vi "testevent.vi"() -> ()   [LabVIEW 2011]
panel:
  out "Time":u32
  in  "stop":bool
  out "Beam2 Far_2>>XHair":u16(ring)
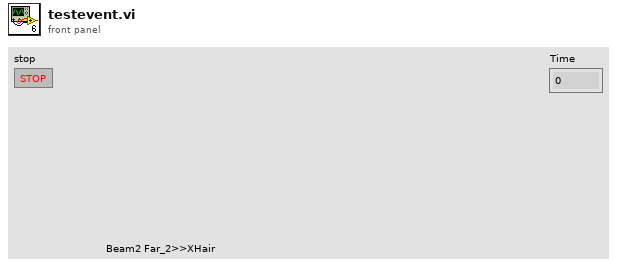
[diagram p1: front panel]
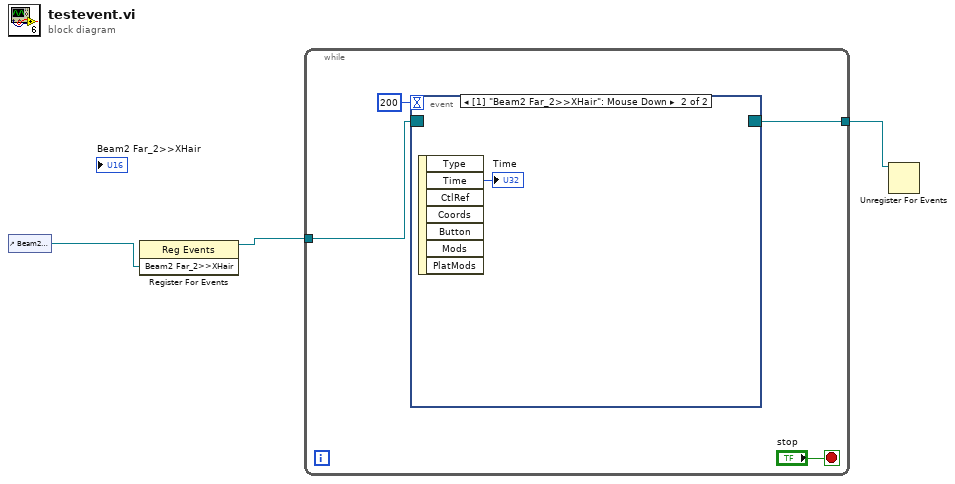
[diagram p0: block diagram]
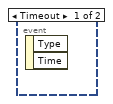
[diagram p2: hidden frame]
diagram:
  n1 = control-ref of="Beam2 Far_2>>XHair"() -> (w3:refnum<vi>)
  n2 = register-events(w3) -> (reference out=w2:refnum<event-registration>)  [unwired: 2 in, 1 out]
  n3 = while {
    tunnel: w2 -> [w5]
    tunnel: [w4] -> w1
    stop <- "stop" stop-if-true
    n4 = event shown="[1] \"Beam2 Far_2>>XHair\": Mouse Down" {
      selector: w5 -> [_ _]
      dyn-events: [_ _] -> w4
      timeout: 200 -> [_ _]
      event Timeout {
        n5 = event-data() -> ()  [unwired: 1 in, 2 out]
      }
      event "Beam2 Far_2>>XHair": Mouse Down {
        n6 = event-data() -> ("Time"=→"Time":u32)  [unwired: 1 in, 6 out]
      }
    }
  }
  n7 = Unregister For Events(event registration refnum=w1) -> ()  [unwired: 1 in, 1 out]
